vi "Fc_MenuSelections.vi"(6 "Cluster References":T2, 7 "ItemTag":string, 8 "error in (no error)":errorcluster, 9 "Cluster in":T1, 10 "VI caller":refnum<vi>, 11 "WaveformGraph in":refnum<vi>) -> (0 "error out":errorcluster, 3 "Cluster out":T1)   [LabVIEW 2022 SP3]
doc: "This function is used to select possible selection in the current window plot."
uses:
  <vilib>/Analysis/1siggen.llb/Ramp Pattern by Samples.vi
  <vilib>/Analysis/NI_AALBase.lvlib
  <vilib>/gmath/NI_Gmath.lvlib
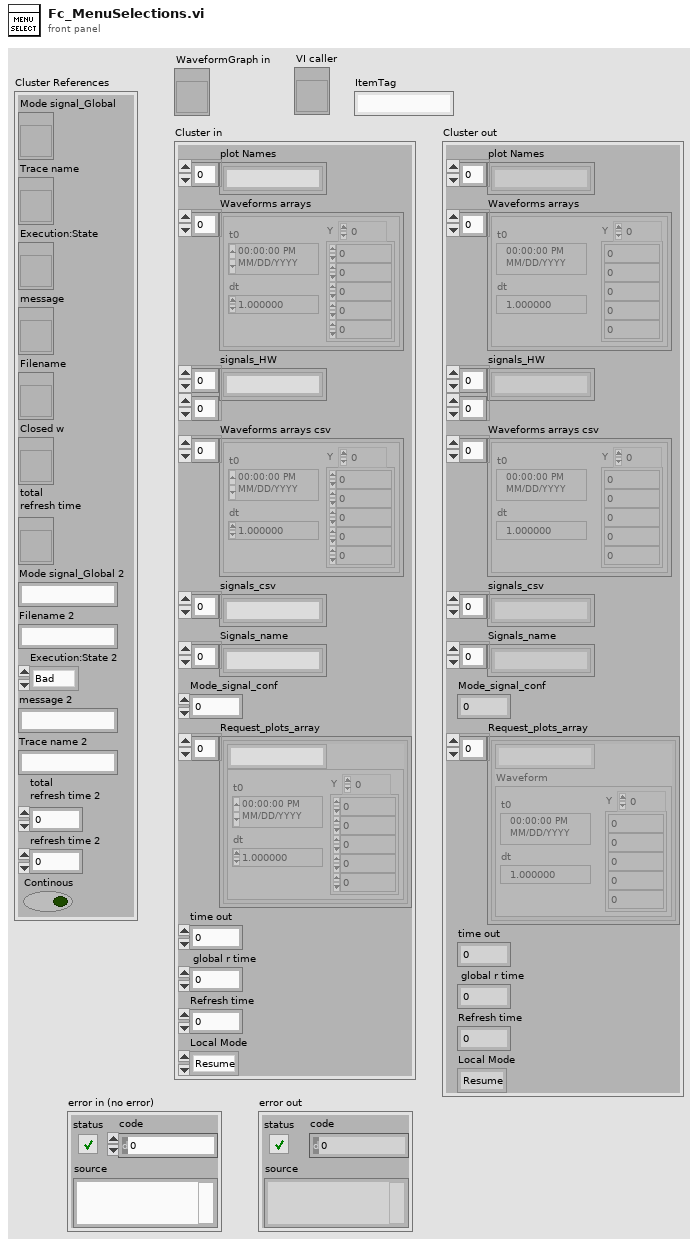
[diagram p1: front panel]
types:
  T1 = cluster{"plot Names":string[], "Waveforms arrays":waveform(dbl)[], "signals_HW":string[][], "Waveforms arrays csv":waveform(dbl)[], "signals_csv":string[], "Signals_name":string[], "Mode_signal_conf":u8, "Request_plots_array":cluster{string, "Waveform":waveform(dbl)}[], "time out":i32, " global r time":u32, "Refresh time":u32, "Local Mode":enum32{"Resume", "Hold"}}
  T2 = cluster{"Mode signal_Global":refnum<vi>, "Trace name":refnum<vi>, "Execution:State":refnum<vi>, "message":refnum<vi>, "Filename":refnum<vi>, "Closed w":refnum<vi>, "total \nrefresh time":refnum<vi>, "Mode signal_Global 2":string, "Filename 2":string, "Execution:State 2":enum32{"Bad", "Idle", "Run top level", "Running"}, "message 2":string, "Trace name 2":string, "total \nrefresh time 2":i32, "refresh time 2":i32, "Continous":bool}
  T3 = enum32{"Bad", "Idle", "Run top level", "Running"}
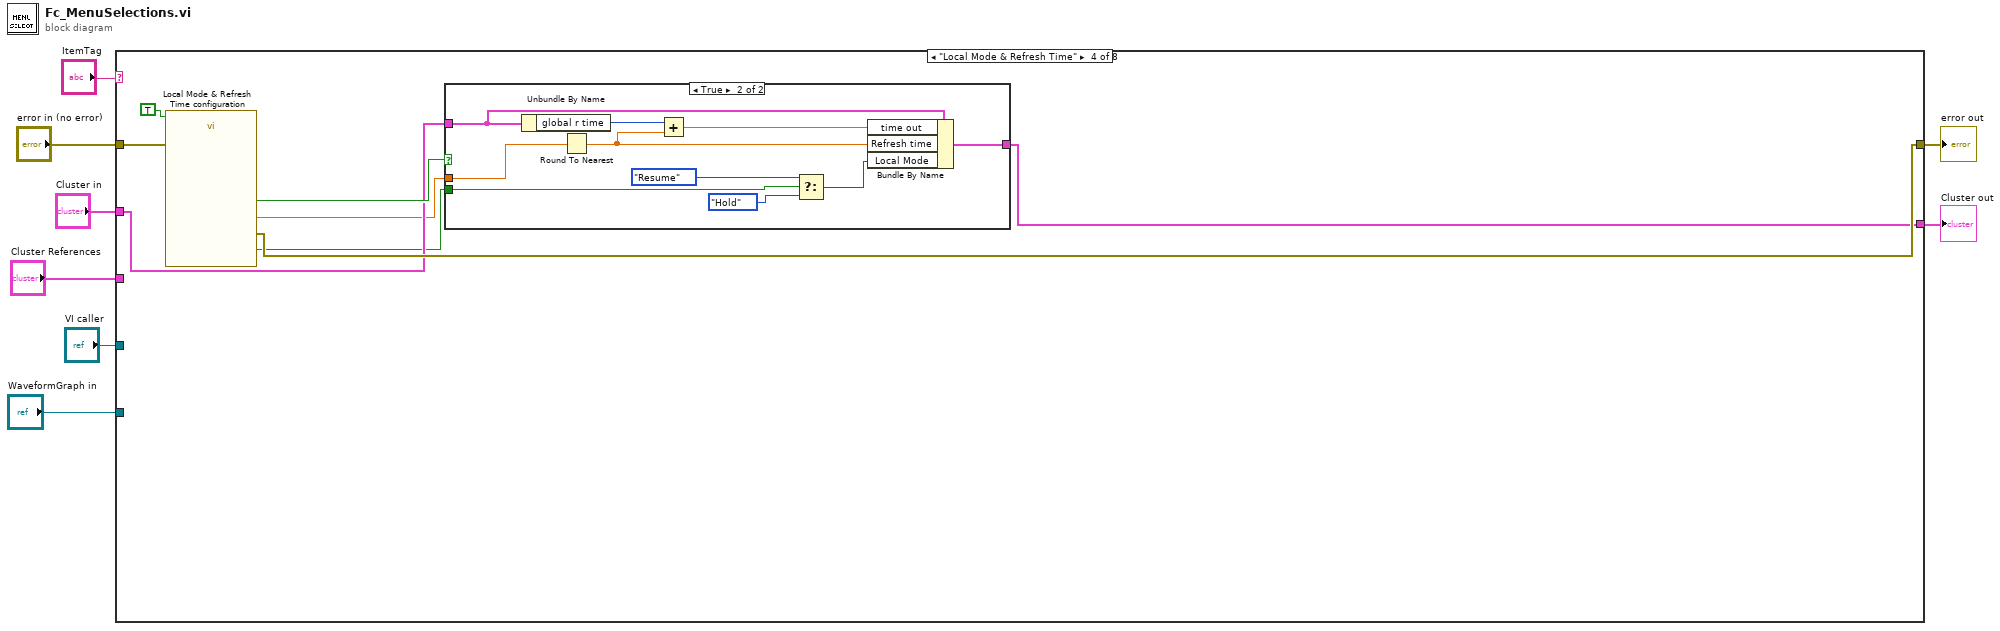
[diagram p0: block diagram]
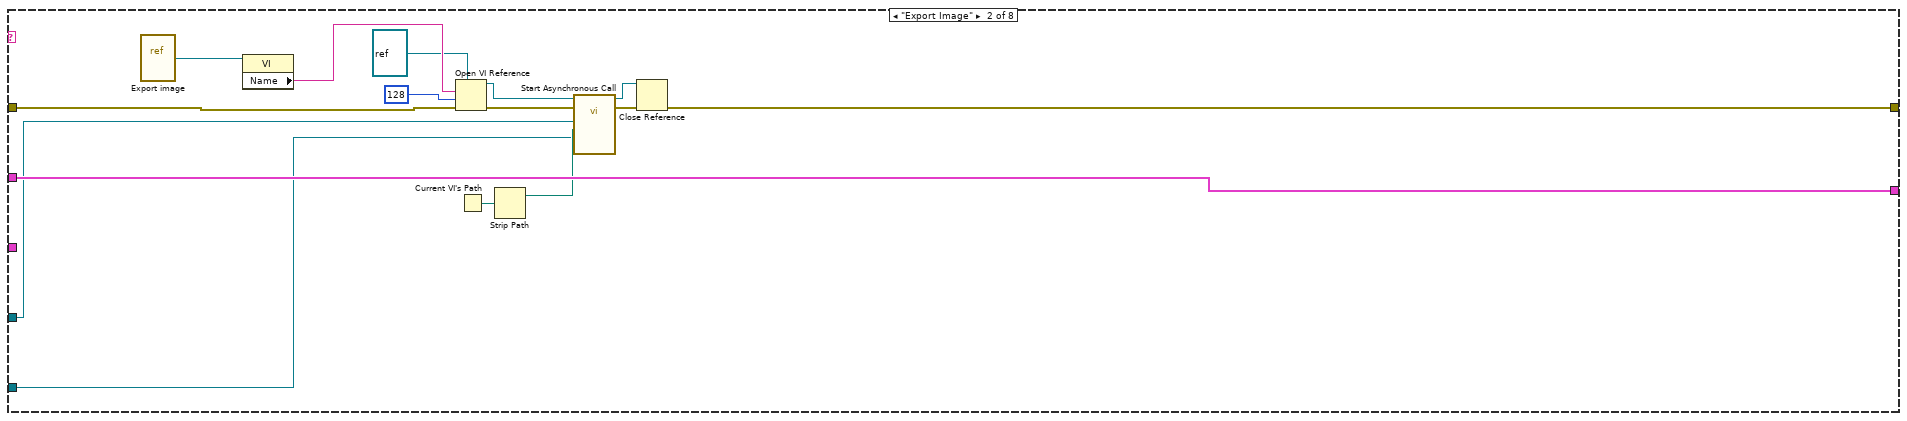
[diagram p3: hidden frame]
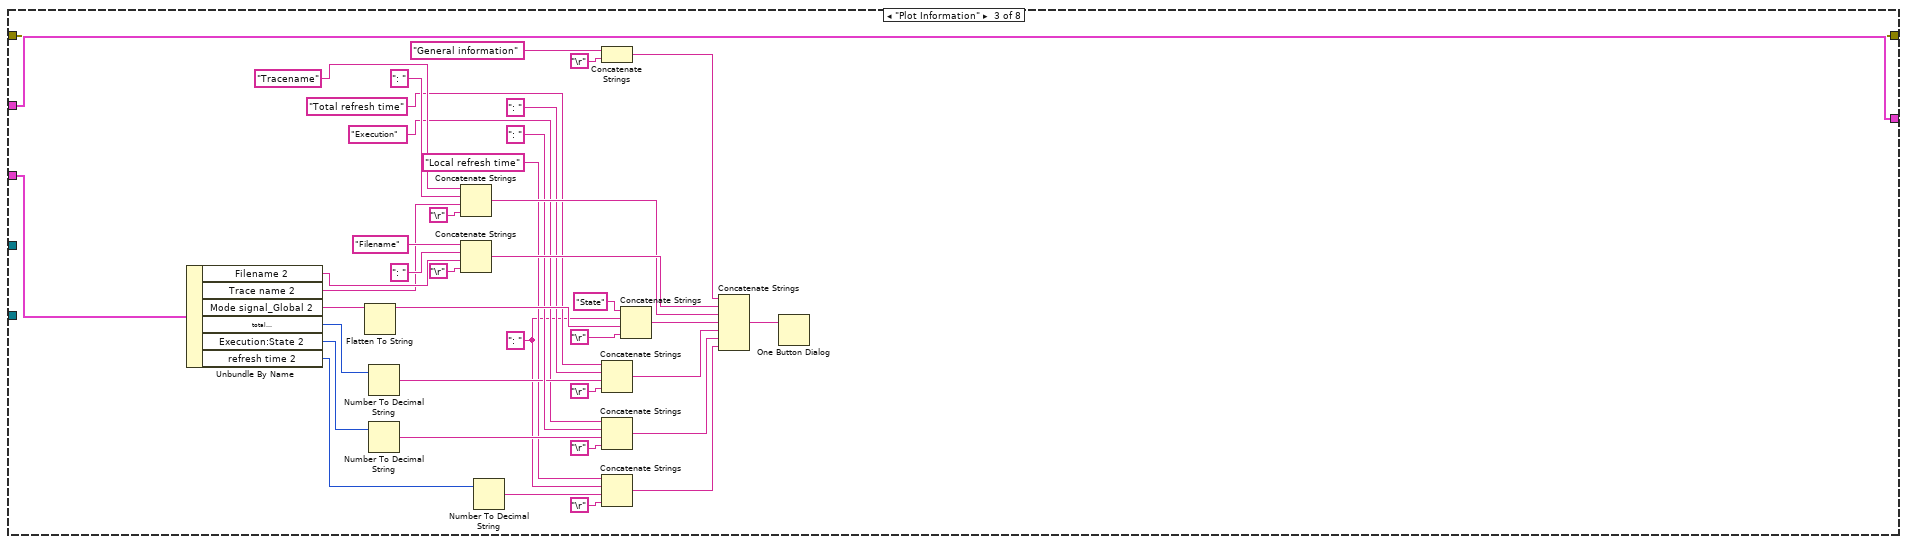
[diagram p4: hidden frame]
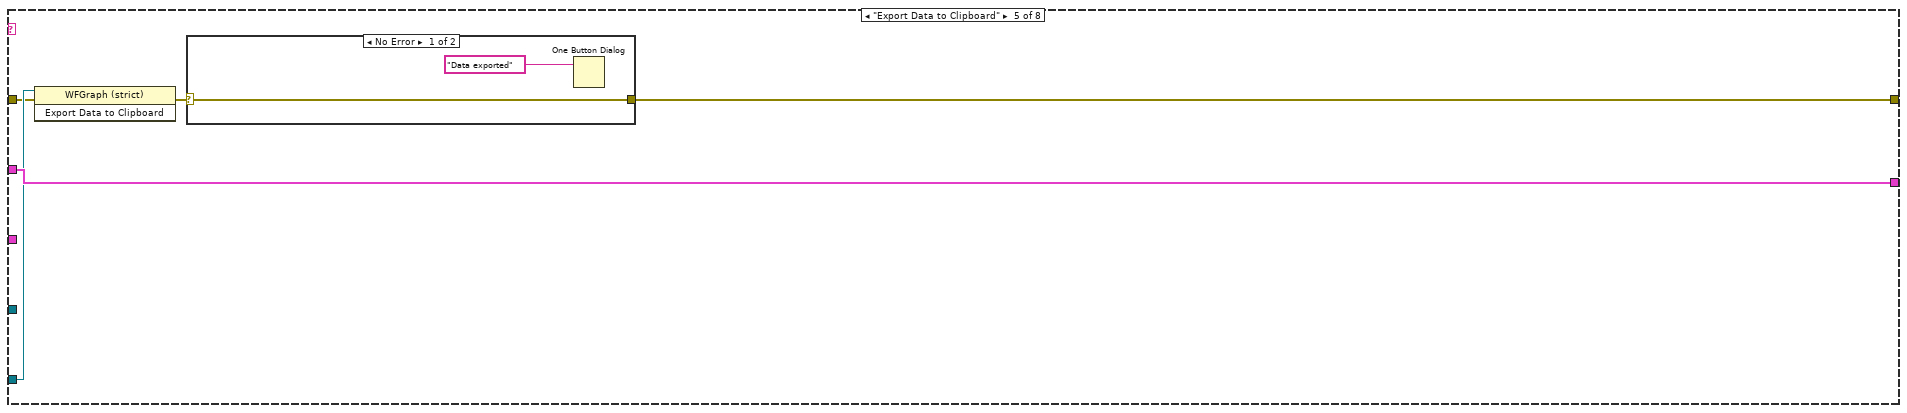
[diagram p6: hidden frame]
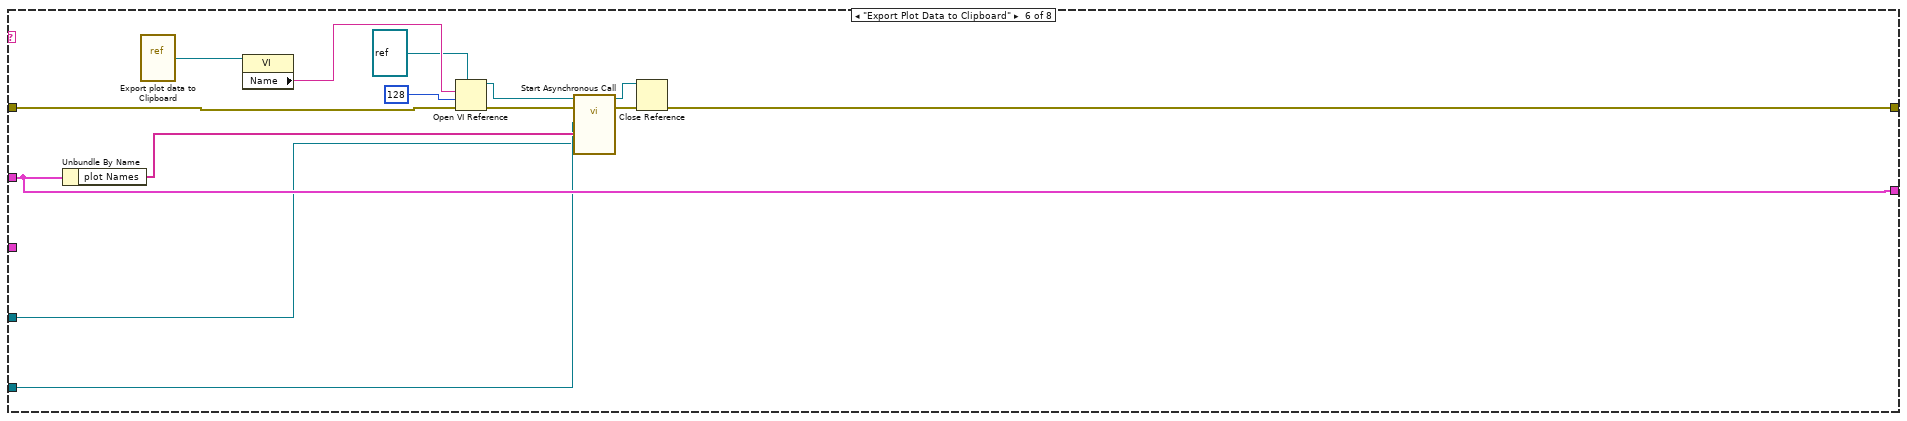
[diagram p8: hidden frame]
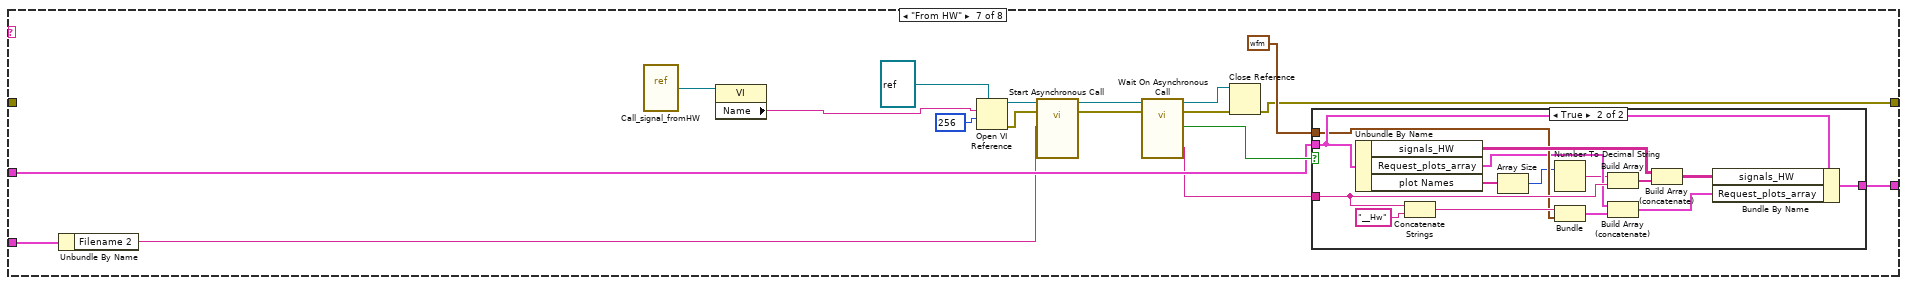
[diagram p9: hidden frame]
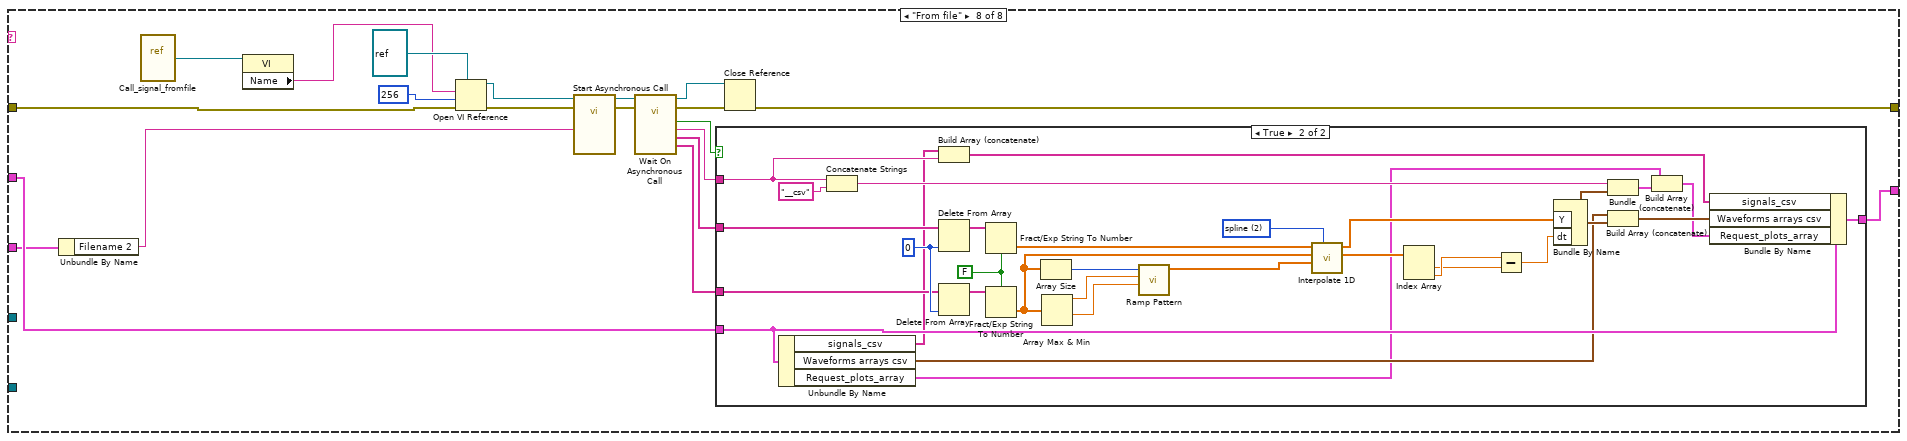
[diagram p11: hidden frame]
diagram:
  n1 = case shown="\"Local Mode & Refresh Time\"" "ItemTag" {
    tunnel: [w10 w25 w65 w67 w89 w100 w120 w154] -> w4
    tunnel: "Cluster in" -> [w10 w25 w65 w69 w89 w100 w112 w155]
    tunnel: [w9 w14 w64 w71 w88 w96 w109 w144] -> w5
    tunnel: "error in (no error)" -> [w9 w13 w64 w72 w85 w95 _ w143]
    tunnel: "WaveformGraph in" -> [_ w12 _ _ w87 w94 _ _]
    tunnel: "VI caller" -> [_ w11 _ _ _ w93 _ _]
    tunnel: "Cluster References" -> [_ _ w63 _ _ _ w107 w142]
    frame "False", Default {
    }
    frame "Export Image" {
      n2 = vi-ref "Export image.vi"() -> (w19:refnum<vi>)
      n3 = property class="VI"(reference=w19) -> ("Name"=w21:string)  [unwired: 1 in, 2 out]
      n4 = Open VI Reference(type specifier VI Refnum (for type only)=refnum<vi> refnum ("reference"), vi path=w21, options=128, error in (no error)=w13) -> (vi reference=w22:refnum<vi>, error out=w23:errorcluster)  [unwired: 2 in]
      n5 = Current VI's Path() -> (path=w24:path)
      n6 = Strip Path(path=w24) -> (stripped path=w17:path)  [unwired: 1 out]
      n7 = call-by-ref "Start Asynchronous Call"(reference=w22, error in=w23, "Graph reference"=w12, "Folder selection"=w17, "VI caller"=w11) -> (reference out=w16:refnum<vi>, error out=w15:errorcluster)  [unwired: 8 in, 1 out]
      n8 = Close Reference(reference=w16, error in (no error)=w15) -> (error out=w14:errorcluster)
    }
    frame "Plot Information" {
      w27 = ": " ("string")
      n9 = Unbundle By Name(w63) -> ("Filename 2"=w40:string, "Trace name 2"=w39:string, "Mode signal_Global 2"=w37:string, "total \nrefresh time 2"=w35:i32, "Execution:State 2"=w33:T3, "refresh time 2"=w29:i32)
      n10 = Flatten To String(anything=w37) -> (data string=w54:string)  [unwired: 3 in, 2 out]
      n11 = Number To Decimal String(number=w35) -> (decimal integer string=w34:string)  [unwired: 1 in]
      n12 = Number To Decimal String(number=w33) -> (decimal integer string=w47:string)  [unwired: 1 in]
      n13 = Concatenate Strings("Tracename" ("string"), ": " ("string"), w39, "\r") -> (w57:string)
      n14 = Concatenate Strings("Filename" ("string"), ": " ("string"), w40, "\r") -> (w58:string)
      n15 = Number To Decimal String(number=w29) -> (decimal integer string=w31:string)  [unwired: 1 in]
      n16 = Concatenate Strings("General information" ("string"), "\r") -> (w42:string)
      n17 = Concatenate Strings("Total refresh time" ("string"), ": " ("string"), w34, "\r") -> (w50:string)
      n18 = Concatenate Strings("Execution" ("string"), ": " ("string"), w47, "\r") -> (w46:string)
      n19 = Concatenate Strings("Local refresh time" ("Label.Text"), w27, w31, "\r") -> (w26:string)
      n20 = Concatenate Strings("State" ("Label.Text"), w27, w54, "\r") -> (w53:string)
      n21 = Concatenate Strings(w42, w58, w57, w53, w50, w46, w26) -> (w45:string)
      n22 = One Button Dialog(message=w45) -> ()  [unwired: 1 in, 1 out]
    }
    frame "Local Mode & Refresh Time" {
      n23 = call "Local Mode & Refresh Time configuration"("Enable"=TRUE, "error in (no error)"=w72) -> ("Refresh time"=w68:dbl, "Resume getting data"=w66:bool, "OK"=w70:bool, "error out"=w71:errorcluster)  [unwired: 14 in]
      n24 = case shown="True" w70 {
        tunnel: w69 -> [w74 w80]
        tunnel: w68 -> [_ w83]
        tunnel: [w74 w79] -> w67
        tunnel: w66 -> [_ w78]
        frame False {
        }
        frame True {
          n25 = Unbundle By Name(w80) -> ("global r time"=w84:u32)
          n26 = Round To Nearest(number=w83) -> (nearest integer value=w82:dbl)
          n27 = Add(x=w84, y=w82) -> (x+y=w81:dbl)
          n28 = Select(t=enum32{"Resume", "Hold"}."Resume" ("Local Mode"), s=w78, f=enum32{"Resume", "Hold"}."Hold" ("Local Mode")) -> (s? t:f=w75:enum32{"Resume", "Hold"})
          n29 = Bundle By Name(cluster=w80, "time out"=w81, "Refresh time"=w82, "Local Mode"=w75) -> (w79:T1)
        }
      }
    }
    frame "Export Data to Clipboard" {
      n30 = invoke class="WFGraph (strict)" method="Export Data to Clipboard"(reference=w87, error in=w85) -> (error out=w86:errorcluster)  [unwired: 1 in, 2 out]
      n31 = case shown="No Error" w86 {
        selector: w86 -> [w90 w92]
        tunnel: [w90 w92] -> w88
        frame No Error {
          n32 = One Button Dialog(message="Data exported") -> ()  [unwired: 1 in, 1 out]
        }
        frame Error {
        }
      }
    }
    frame "Export Plot Data to Clipboard" {
      n33 = Unbundle By Name(w100) -> ("plot Names"=w102:string[])
      n34 = vi-ref "Export plot data to Clipboard.vi"() -> (w97:refnum<vi>)
      n35 = property class="VI"(reference=w97) -> ("Name"=w106:string)  [unwired: 1 in, 2 out]
      n36 = Open VI Reference(type specifier VI Refnum (for type only)=refnum<vi> refnum ("reference"), vi path=w106, options=128, error in (no error)=w95) -> (vi reference=w105:refnum<vi>, error out=w104:errorcluster)  [unwired: 2 in]
      n37 = call-by-ref "Start Asynchronous Call"(reference=w105, error in=w104, "VI caller"=w93, "List Plots"=w102, "Graph reference"=w94) -> (reference out=w99:refnum<vi>, error out=w98:errorcluster)  [unwired: 2 in, 1 out]
      n38 = Close Reference(reference=w99, error in (no error)=w98) -> (error out=w96:errorcluster)
    }
    frame "From HW" {
      n39 = Unbundle By Name(w107) -> ("Filename 2"=w108:string)
      n40 = vi-ref "Call_signal_fromHW.vi"() -> (w121:refnum<vi>)
      n41 = property class="VI"(reference=w121) -> ("Name"=w113:string)  [unwired: 1 in, 2 out]
      n42 = Open VI Reference(type specifier VI Refnum (for type only)=refnum<vi> refnum ("reference"), vi path=w113, options=256) -> (vi reference=w122:refnum<vi>, error out=w124:errorcluster)  [unwired: 3 in]
      n43 = call-by-ref "Start Asynchronous Call"(reference=w122, error in=w124, "Plot window"=w108) -> (reference out=w118:refnum<vi>, error out=w119:errorcluster)  [unwired: 2 in, 3 out]
      n44 = call-by-ref "Wait On Asynchronous Call"(reference=w118, error in=w119) -> (reference out=w117:refnum<vi>, error out=w116:errorcluster, "Y name"=w110:string, "Ready?"=w115:bool)  [unwired: 3 in, 1 out]
      n45 = Close Reference(reference=w117, error in (no error)=w116) -> (error out=w109:errorcluster)
      n46 = case shown="True" w115 {
        tunnel: w110 -> [_ w139]
        tunnel: [w125 w134] -> w120
        tunnel: w112 -> [w125 w138]
        tunnel: waveform(dbl) {"t0"=timestamp(0 s since 1904-01-01), "dt"=1.0, "Y"=[]} ("Waveform") -> [_ w132]
        frame False {
        }
        frame True {
          n47 = Unbundle By Name(w138) -> ("signals_HW"=w137:string[][], "Request_plots_array"=w131:cluster{string, "Waveform":waveform(dbl)}[], "plot Names"=w128:string[])
          n48 = Concatenate Strings(w139, "__Hw" ("string")) -> (w133:string)
          n49 = Array Size(array=w128) -> (size(s)=w127:i32)
          n50 = Number To Decimal String(number=w127) -> (decimal integer string=w126:string)  [unwired: 1 in]
          n51 = Bundle(w133, "Waveform"=w132) -> (w130:cluster{string, "Waveform":waveform(dbl)})  [unwired: 1 in]
          n52 = Build Array(w126, w139) -> (w136:string[])
          n53 = Build Array (concatenate)(w131, w130) -> (w129:cluster{string, "Waveform":waveform(dbl)}[])
          n54 = Build Array (concatenate)(w137, w136) -> (w135:string[][])
          n55 = Bundle By Name(cluster=w138, "signals_HW"=w135, "Request_plots_array"=w129) -> (w134:T1)
        }
      }
    }
    frame "From file" {
      n56 = Unbundle By Name(w142) -> ("Filename 2"=w141:string)
      n57 = vi-ref "Call_signal_fromfile.vi"() -> (w158:refnum<vi>)
      n58 = property class="VI"(reference=w158) -> ("Name"=w152:string)  [unwired: 1 in, 2 out]
      n59 = Open VI Reference(type specifier VI Refnum (for type only)=refnum<vi> refnum, vi path=w152, options=256, error in (no error)=w143) -> (vi reference=w156:refnum<vi>, error out=w160:errorcluster)  [unwired: 2 in]
      n60 = call-by-ref "Start Asynchronous Call"(reference=w156, error in=w160, "Plot window"=w141) -> (reference out=w153:refnum<vi>, error out=w151:errorcluster)  [unwired: 3 in, 4 out]
      n61 = call-by-ref "Wait On Asynchronous Call"(reference=w153, error in=w151) -> (reference out=w146:refnum<vi>, error out=w145:errorcluster, "Y subarray"=w147:string[], "X subarray"=w148:string[], "Curve name"=w149:string, "Ready?"=w150:bool)  [unwired: 4 in]
      n62 = case shown="True" w150 {
        tunnel: w148 -> [_ w191]
        tunnel: w147 -> [_ w190]
        tunnel: w149 -> [_ w173]
        tunnel: w155 -> [w161 w167]
        tunnel: [w161 w168] -> w154
        frame False {
        }
        frame True {
          w182 = 2 items=["nearest", "linear", "spline", "cubic Hermite", "Lagrange"] ("method")
          w187 = FALSE ("use system decimal point (T)")
          w192 = 0 ("index")
          n63 = Unbundle By Name(w167) -> ("signals_csv"=w165:string[], "Waveforms arrays csv"=w166:waveform(dbl)[], "Request_plots_array"=w164:cluster{string, "Waveform":waveform(dbl)}[])
          n64 = Concatenate Strings(w173, "__csv" ("string")) -> (w172:string)
          n65 = Build Array (concatenate)(w165, w173) -> (w170:string[])
          n66 = Delete From Array(array=w191, index=w192) -> (array with subset deleted=w188:string[])  [unwired: 1 in, 1 out]
          n67 = Delete From Array(array=w190, index=w192) -> (array with subset deleted=w189:string[])  [unwired: 1 in, 1 out]
          n68 = Fract/Exp String To Number(use system decimal point (T)=w187, string=w188) -> (number=w179:dbl[])  [unwired: 2 in, 1 out]
          n69 = Fract/Exp String To Number(use system decimal point (T)=w187, string=w189) -> (number=w181:dbl[])  [unwired: 2 in, 1 out]
          n70 = Array Size(array=w181) -> (size(s)=w185:i32)
          n71 = Array Max & Min(array=w181) -> (max value=w184:dbl, min value=w183:dbl)  [unwired: 2 out]
          n72 = call-poly <vilib>:"Ramp Pattern.vi"("start"=w183, "end"=w184, "samples"=w185) -> ("Ramp Pattern"=w180:dbl[])  [unwired: 7 in, 1 out]
          n73 = call <vilib>:"Interpolate 1D.vi"("method"=w182, "xi"=w180, "X"=w181, "Y"=w179) -> ("xi used"=w178:dbl[], "yi"=w177:dbl[])  [unwired: 5 in, 1 out]
          n74 = Index Array(array=w178) -> (element #1=w175:dbl, element #2=w176:dbl)  [unwired: 2 in]
          n75 = Subtract(x=w176, y=w175) -> (x-y=w174:dbl)
          n76 = Bundle By Name("Y"=w177, "dt"=w174) -> (w171:waveform(dbl))  [unwired: 1 in]
          n77 = Bundle(w172, w171) -> (w163:cluster{string, waveform(dbl)})  [unwired: 1 in]
          n78 = Build Array (concatenate)(w166, w171) -> (w169:waveform(dbl)[])
          n79 = Build Array (concatenate)(w164, w163) -> (w162:cluster{string, "Waveform":waveform(dbl)}[])
          n80 = Bundle By Name(cluster=w167, "signals_csv"=w170, "Waveforms arrays csv"=w169, "Request_plots_array"=w162) -> (w168:T1)
        }
      }
      n81 = Close Reference(reference=w146, error in (no error)=w145) -> (error out=w144:errorcluster)
    }
  }
  "error out" <- w5
  "Cluster out" <- w4
